vi "数值控件介绍.vi"() -> ()   [LabVIEW 2018]
panel:
  out "数字(0-1)":dbl
  out "x^2":dbl
  in  "x":dbl
  out "x+y":dbl
  in  "加数2":dbl
  in  "加数1":dbl
  out "液罐":dbl(slide) scale=0.0..10.0
  in  "量表 2":dbl(knob) scale=0.0..10.0
  out "量表":dbl(knob) scale=0.0..10.0
  in  "数值 3":dbl min=0.0 max=10.0 step=1.0
  out "仪表":dbl(knob) scale=0.0..10.0
  in  "滑动杆":dbl(slide) scale=0.0..10.0
  out "数值 2":dbl
  in  "数值":dbl min=0.0 max=10.0
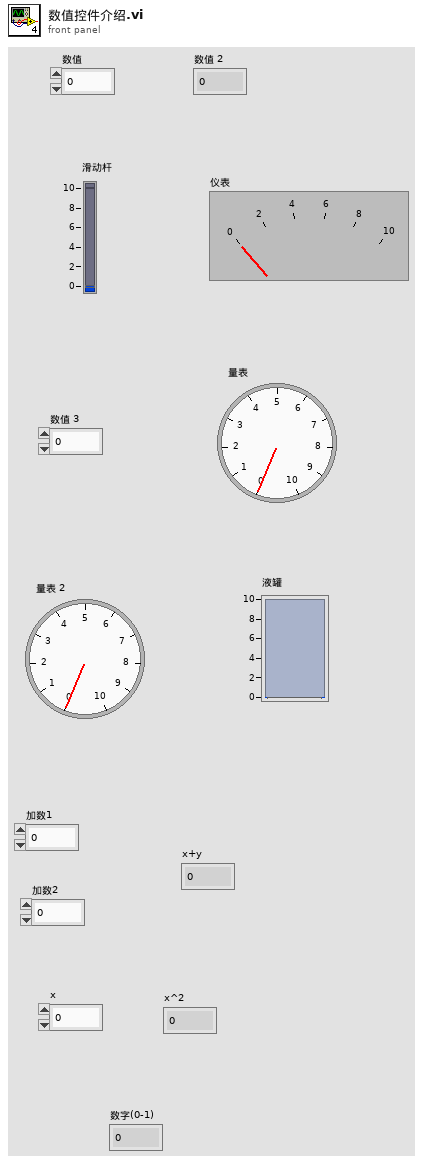
[diagram p1: front panel]
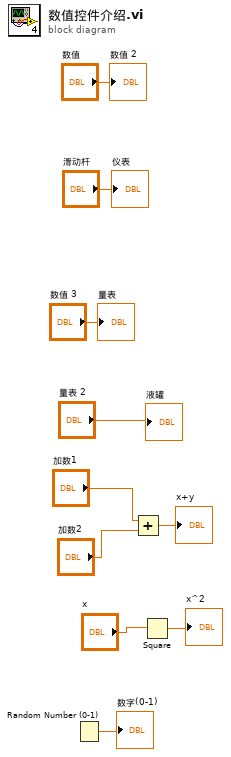
[diagram p0: block diagram]
diagram:
  n1 = Random Number (0-1)() -> (number: 0 to 1=→"数字(0-1)":dbl)
  n2 = Add(x="加数1", y="加数2") -> (x+y=→"x+y":dbl)
  n3 = Square(x="x") -> (x^2=→"x^2":dbl)
  "数值 2" <- "数值"
  "仪表" <- "滑动杆"
  "量表" <- "数值 3"
  "液罐" <- "量表 2"
